vi "Robot Systems 2016.vi"(10 "Robot Commands":T1) -> ()   [LabVIEW 2015]
uses:
  Robot Commands 2016.ctl
  Load SS/Roller State.ctl
  Global Variables/Temp Variables.vi
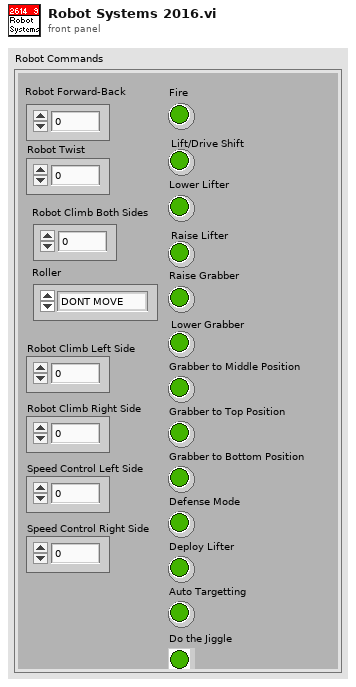
[diagram p1: front panel]
types:
  T1 = typedef "Robot Commands 2016.ctl" = cluster{"Robot Forward-Back":dbl, "Robot Twist":dbl, "Fire":bool, "Lift/Drive Shift":bool, "Raise Lifter":bool, "Raise Grabber":bool, "Lower Grabber":bool, "Roller":T2, "Robot Climb Both Sides":dbl, "Grabber to Middle Position":bool, "Grabber to Top Position":bool, "Grabber to Bottom Position":bool, "Robot Climb Left Side":dbl, "Robot Climb Right Side":dbl, "Speed Control Left Side":dbl, "Speed Control Right Side":dbl, "Lower Lifter":bool, "Defense Mode":bool, "Deploy Lifter":bool, "Auto Targetting":bool, "Do the Jiggle":bool}
  T2 = typedef "Roller State.ctl" = enum16{"DONT MOVE", "Intake", "Outtake"}
  T3 = typedef "Drive Subsystem State.ctl" = enum16{"Drive", "Climb", "Auto Target"}
  T4 = typedef "Ball Gatherer State.ctl" = enum16{"Manual", "Positional"}
  T5 = typedef "Shooter Control.ctl" = enum16{"Enabled", "Disabled"}
  T6 = typedef "Drive Actuator Values Out.ctl" = cluster{"Left Master":dbl, "Right Master":dbl, "Lift/ Drive Shift":bool, "Climb Deploy Motor":dbl, "Deploy Pins":bool}
  T7 = typedef "Load Actuator Values.ctl" = cluster{"Left Grabber Motor":dbl, "Right Grabber Motor":dbl, "Roller Motor":dbl}
  T8 = typedef "Shoot Actuator Values.ctl" = cluster{"Catapult Winch":dbl, "Catapult Solenoid":T9, "Inner LEDs":T9, "Left LEDs":T9, "Right LEDs":T9}
  T9 = typedef "WPI_SolenoidValue.ctl" = enum16{"Off", "On", "Forward", "Reverse"}
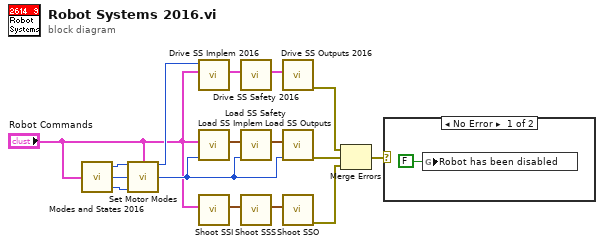
[diagram p0: block diagram]
diagram:
  n1 = call "Modes and States 2016.vi"("Robot Commands"="Robot Commands") -> ("Drive/Climb State"=w6:T3, "Ball Gatherer State"=w2:T4, "Shooter State"=w1:T5)  [unwired: 4 in]
  n2 = call "Set Motor Modes.vi"("Drive/Climb State"=w6, "Robot Commands"="Robot Commands", "Ball Gatherer State"=w2, "Shooter State"=w1) -> ("Drive/Climb State Out"=w5:T3, "Ball Gatherer State Out"=w4:T4)  [unwired: 9 in, 1 out]
  n3 = call "Drive SS Implem 2016.vi"("Robot Commands"="Robot Commands", "Drive/Climb State"=w5) -> ("Drive Actuator Values Out"=w16:T6)  [unwired: 9 in]
  n4 = call "Load SS Implem.vi"("Ball Gatherer State"=w4, "Robot Commands"="Robot Commands") -> ("Load Actuator Values Out"=w14:T7)  [unwired: 9 in]
  n5 = call "Shoot SSI.vi"("Robot Commands"="Robot Commands") -> ("Shoot Actuator Values Out"=w13:T8)  [unwired: 10 in]
  n6 = call "Drive SS Safety 2016.vi"("Drive Actuator Values In"=w16) -> ("Drive Actuator Values Out"=w15:T6)  [unwired: 10 in]
  n7 = call "Load SS Safety.vi"("Ball Gatherer State"=w4, "Load Actuator Values In"=w14) -> ("Load Actuator Values Out"=w11:T7)  [unwired: 9 in]
  n8 = call "Shoot SSS.vi"("Shoot Actuator Values In"=w13) -> ("Shoot Actuator Values Out"=w12:T8)  [unwired: 10 in]
  n9 = call "Drive SS Outputs 2016.vi"("Drive Actuator Values In"=w15) -> ("error out"=w8:errorcluster)  [unwired: 10 in]
  n10 = call "Load SS Outputs.vi"("Ball Gatherer State"=w4, "Load Actuator Values"=w11) -> ("error out"=w10:errorcluster)  [unwired: 9 in]
  n11 = call "Shoot SSO.vi"("Shoot Actuator Values In"=w12) -> ("error out"=w9:errorcluster)  [unwired: 10 in]
  n12 = Merge Errors(w8, w10, w9) -> (w7:errorcluster)
  n13 = case shown="No Error" w7 {
    frame No Error {
      n14 = global write "Temp Variables.vi" "Robot has been disabled"(FALSE ("Robot has been disabled")) -> ()
    }
    frame Error {
    }
  }
